vi "External interactions.vi"(10 "Message":refnum<user-event>, 11 "UUT Result":refnum<user-event>) -> ()   [LabVIEW 2025]
uses:
  Test Unit/UUT Result.ctl
  <vilib>/Test Bench Framework/Test Executive.lvlibp/TestEngine/TestEngine/TestEngine/Typedefs/Report General.ctl
  Full User Interface/Send User Message Argument--cluster.ctl
  Test Unit/Test Unit.lvlib
  Full User Interface/Full User Interface.lvlib
  <vilib>/Test Bench Framework/Test Executive.lvlibp/TestEngine/TestEngine/TestEngine/Test Engine.lvclass
panel:
  in  "Checkbox":bool
  out "当前测试型号":string
  out "General":T1
  in  "设置条码":bool
  in  "启动测试":bool
  out "Error Out":errorcluster
  in  "Error In":errorcluster
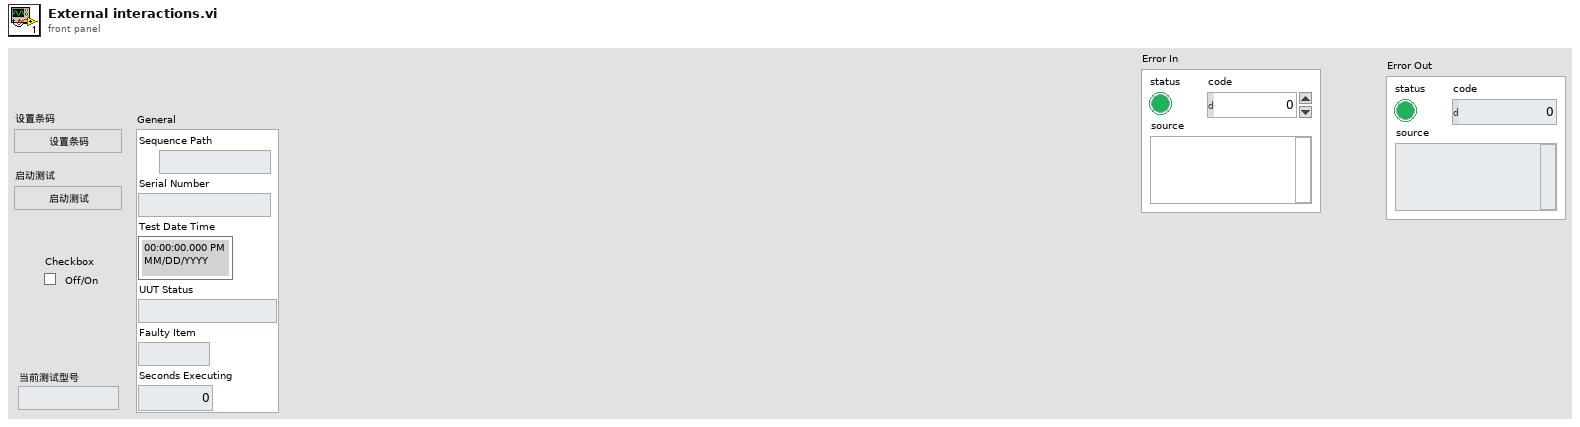
[diagram p1: front panel]
types:
  T1 = typedef "Test Executive.lvlibp/Test Engine.lvlib/Test Engine.lvclass/Report General.ctl" = cluster{"Sequence Path":path, "Serial Number":string, "Test Date Time":timestamp, "UUT Status":string, "Faulty Item":string, "Seconds Executing":dbl}
  T2 = typedef "Full User Interface.lvlib/Send User Message Argument--cluster.ctl" = cluster{"Station ID":i32, "Socket":i32, "UserMessage":string, "MessageData":variant}
  T3 = enum32{"Invalid", "Standard", "Closed", "Hidden", "Minimized", "Maximized"}
  T4 = enum32{"invalid app kind", "Development System", "Run Time System", "Student Edition", "Embedded LabVIEW", "Evaluation", "Custom"}
  T5 = cluster{"Core":cluster{"Current VI Reference":refnum<vi>, "Close Panel on Exit?":bool}, "Your Boolean data":bool, "Your string data":string}
  T6 = cluster{"Current VI Reference":refnum<vi>, "Close Panel on Exit?":bool}
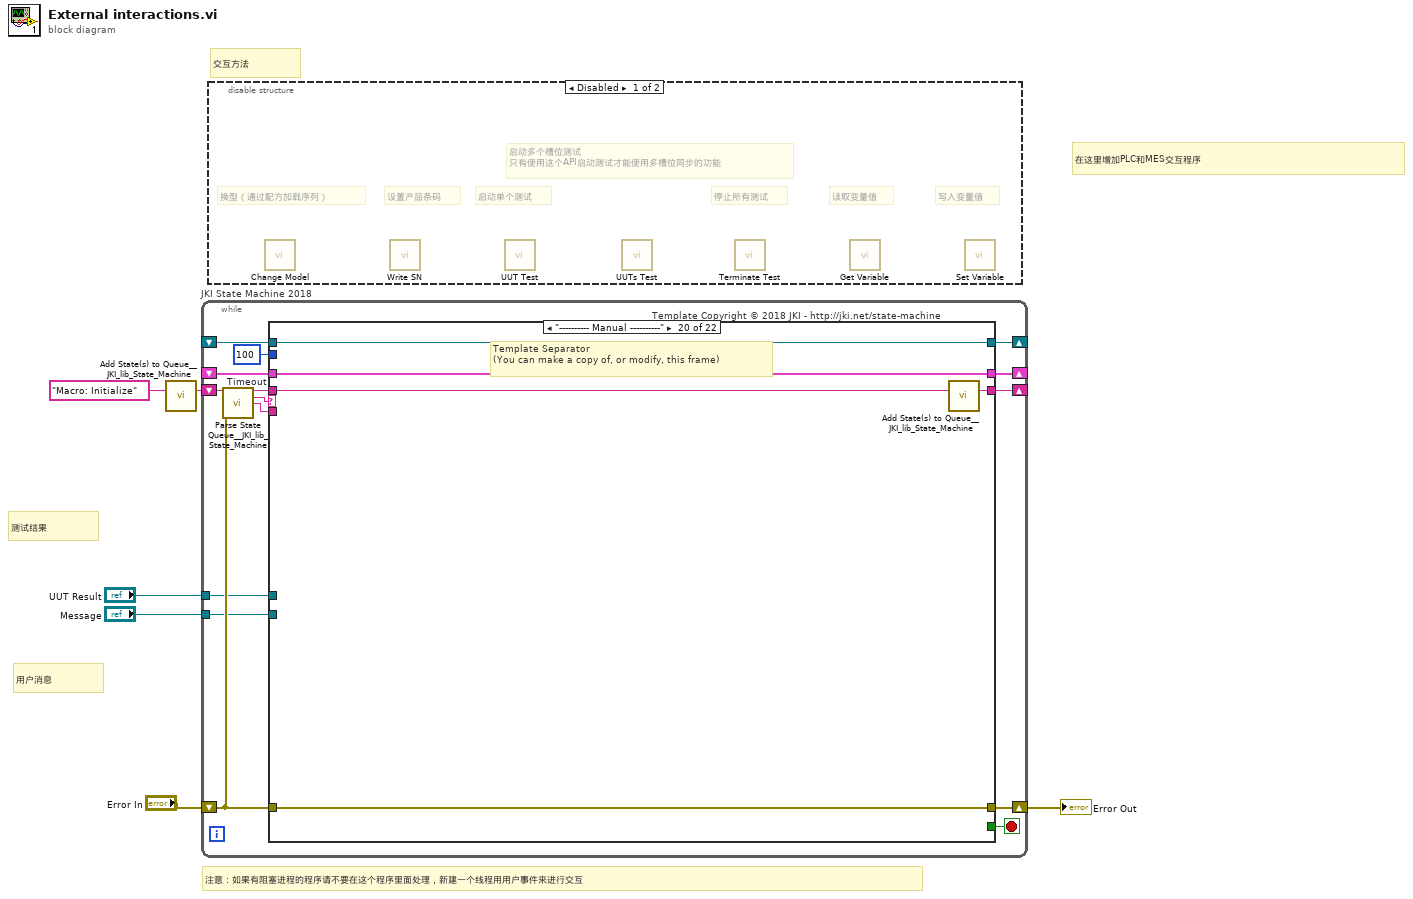
[diagram p0: block diagram]
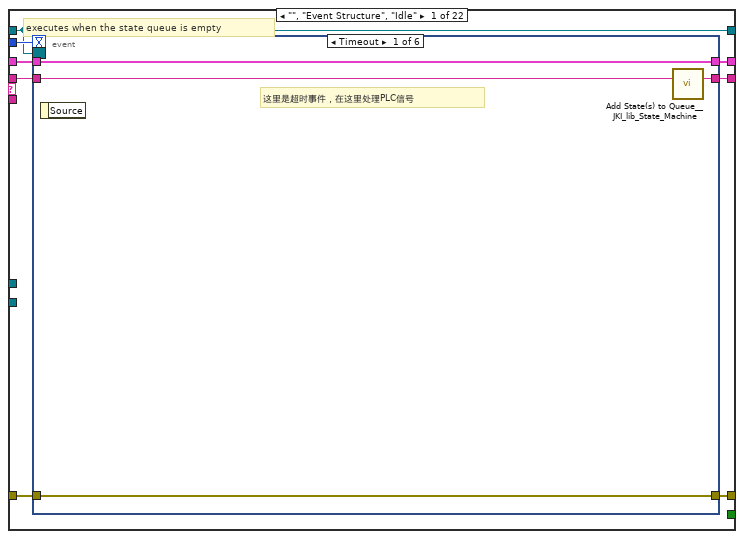
[diagram p2: hidden frame]
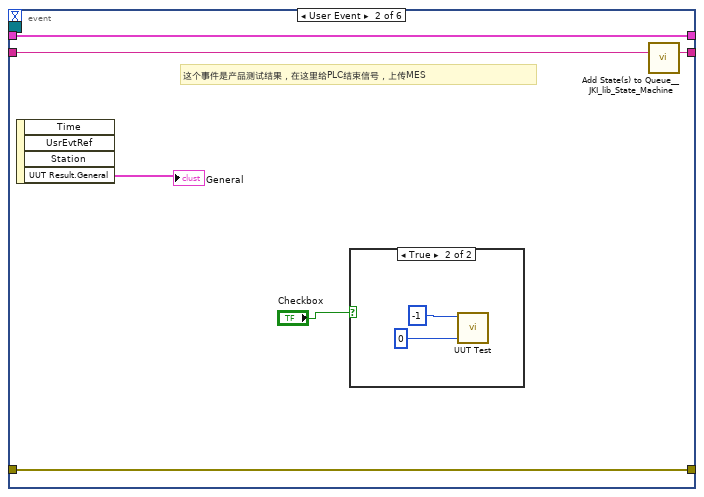
[diagram p3: hidden frame]
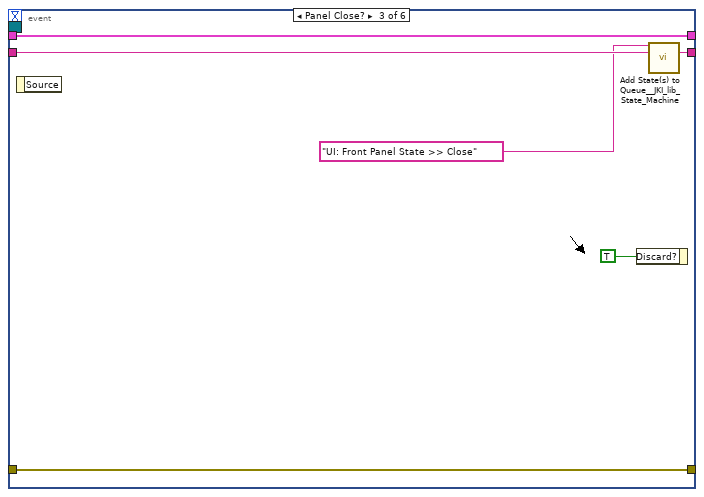
[diagram p5: hidden frame]
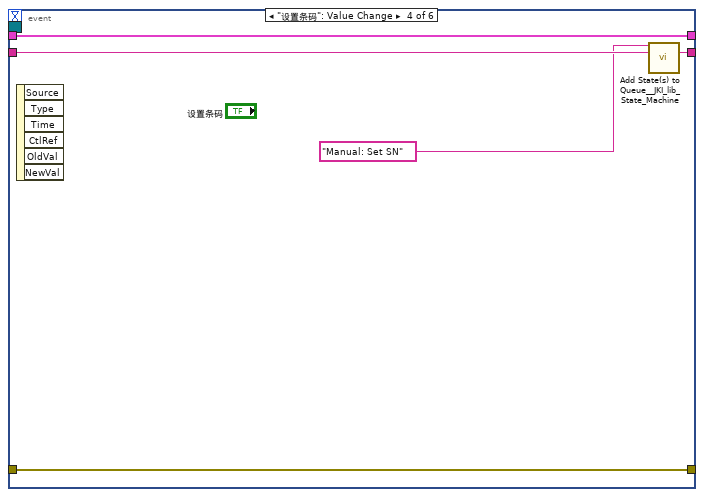
[diagram p6: hidden frame]
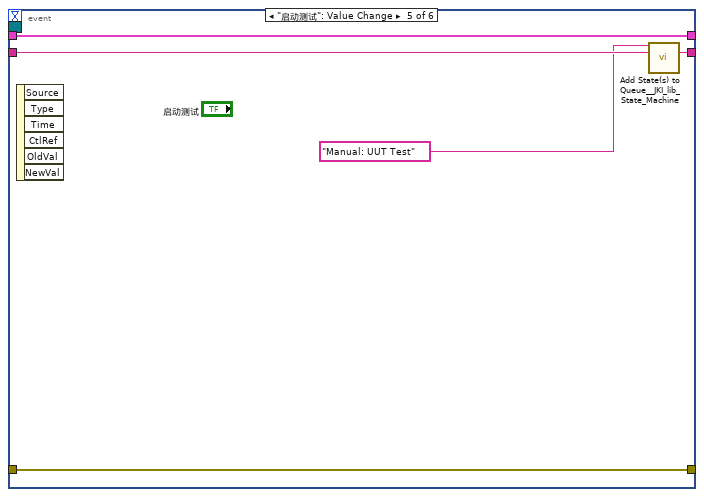
[diagram p7: hidden frame]
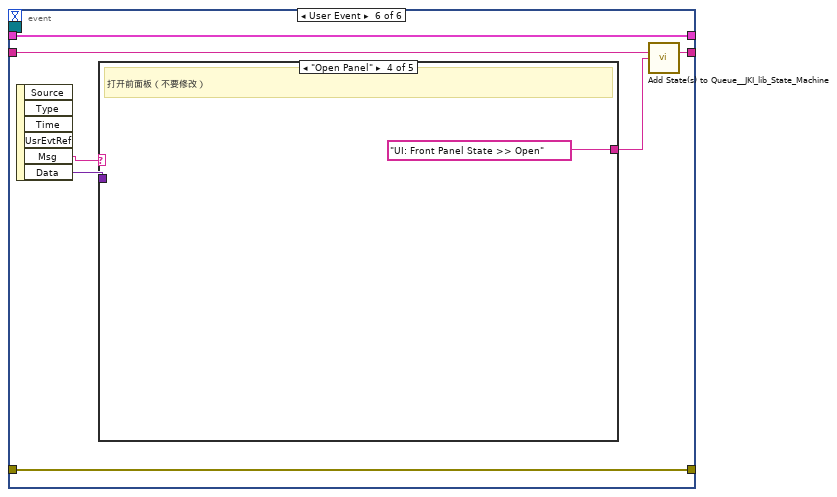
[diagram p8: hidden frame]
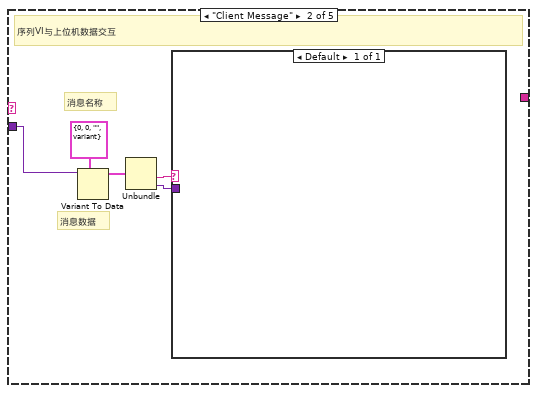
[diagram p10: hidden frame]
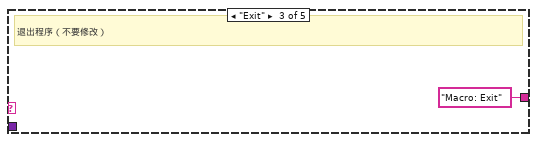
[diagram p11: hidden frame]
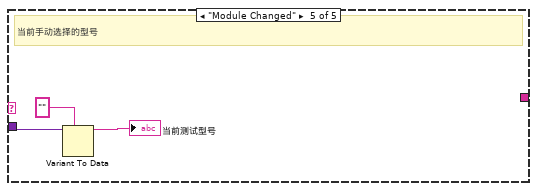
[diagram p12: hidden frame]
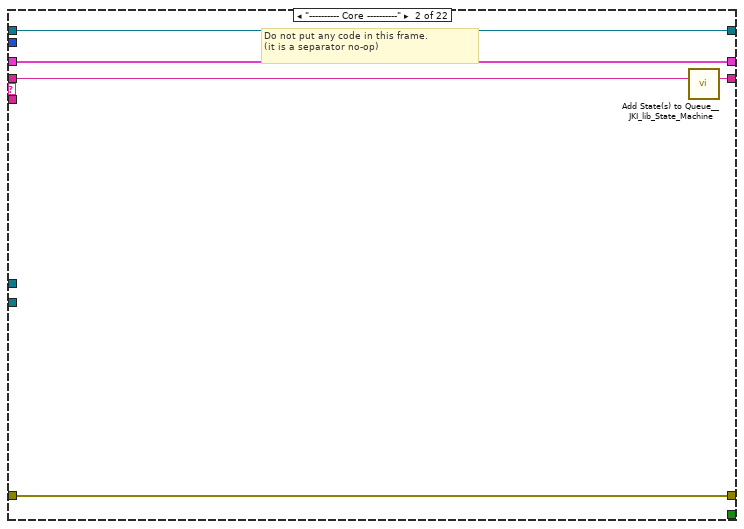
[diagram p13: hidden frame]
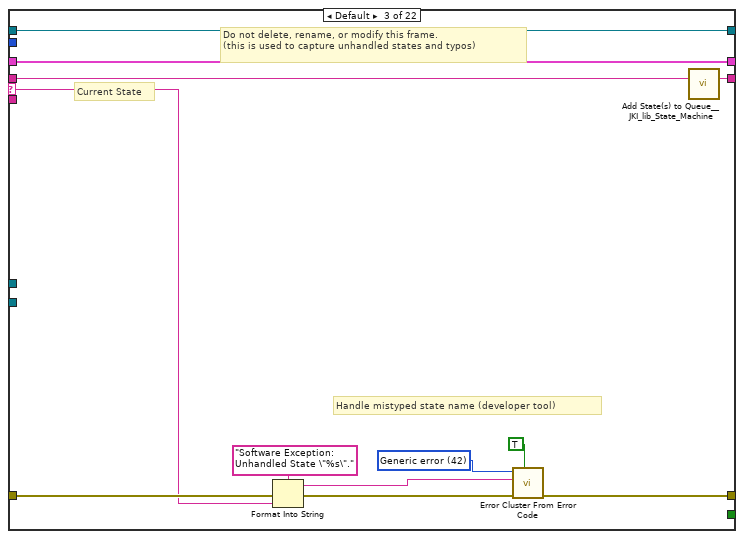
[diagram p14: hidden frame]
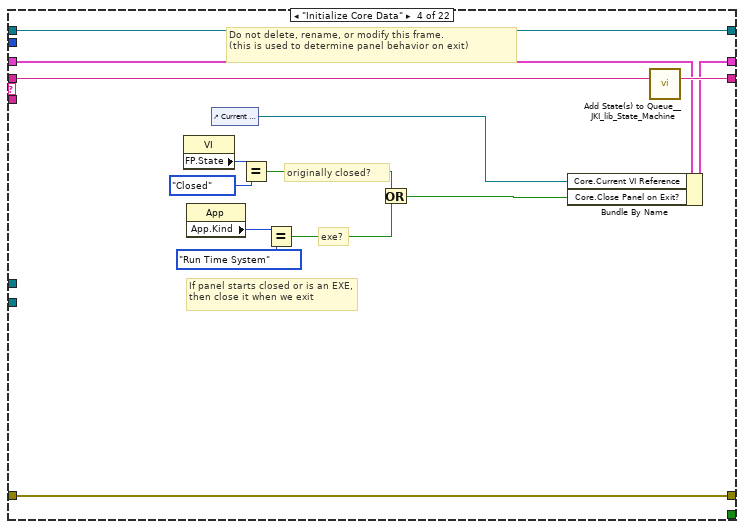
[diagram p15: hidden frame]
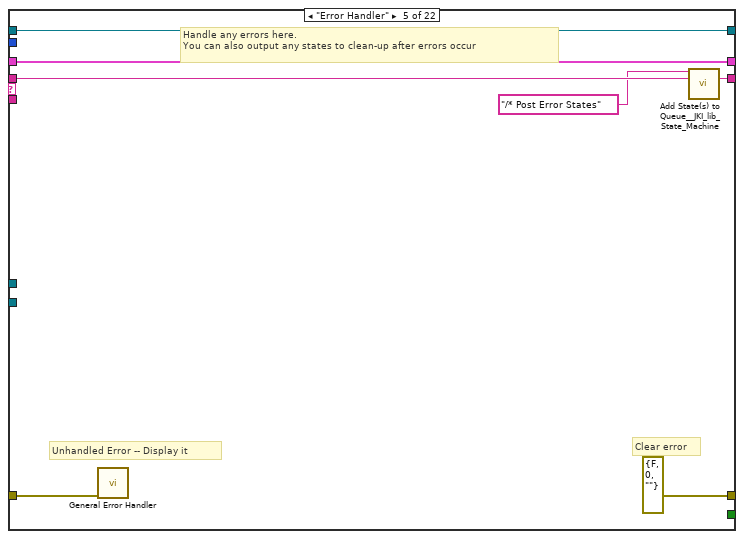
[diagram p16: hidden frame]
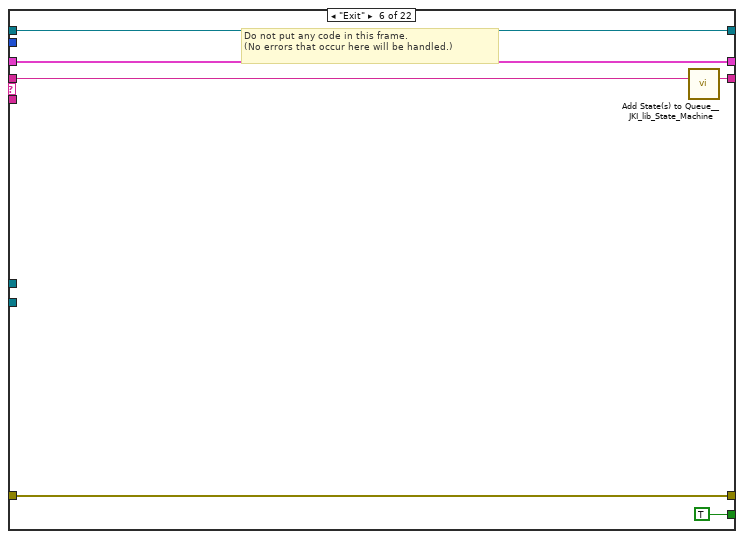
[diagram p17: hidden frame]
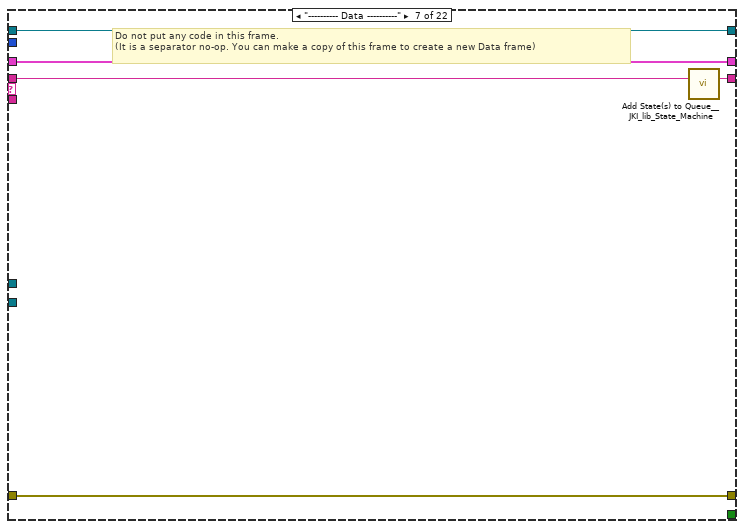
[diagram p18: hidden frame]
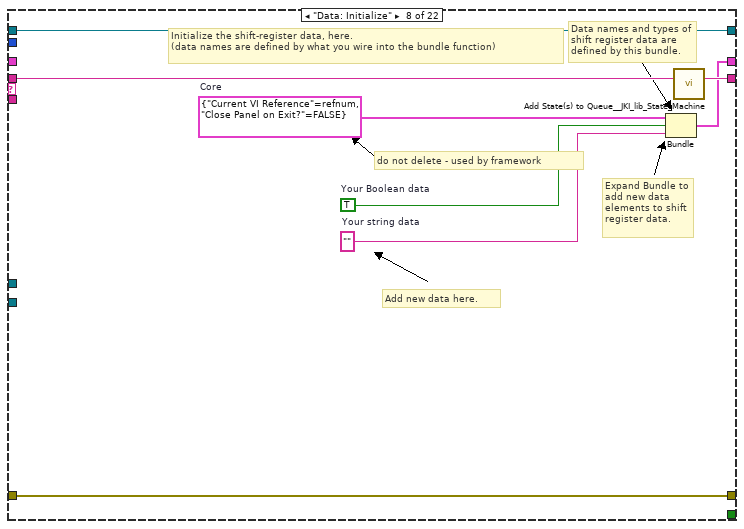
[diagram p19: hidden frame]
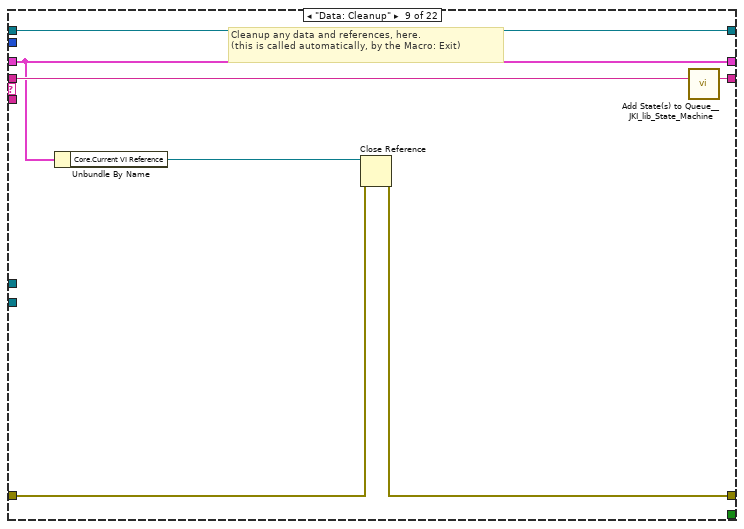
[diagram p20: hidden frame]
diagram:
  # "注意：如果有阻塞进程的程序请不要在这个程序里面处理，新建一个线程用用户事件来进行交互"
  # "在这里增加PLC和MES交互程序"
  # "用户消息"
  # "测试结果"
  # "交互方法"
  n1 = call <vilib>:"Add State(s) to Queue__JKI_lib_State_Machine.vi"("State(s) in (\"\")"="Macro: Initialize") -> ("States Out"=w6:string)  [unwired: 14 in]
  n2 = while "JKI State Machine 2018" {
    shift-right: [w14] -> _
    shift-left: _ -> [w13]
    shift-right: [w17] -> w3
    shift-left: "Error In" -> [w11]
    shift-right: [w16] -> _
    shift-left: w6 -> [w18]
    shift-right: [w10] -> _
    shift-left: _ -> [w9]
    tunnel: "UUT Result" -> [w8]
    tunnel: "Message" -> [w7]
    stop <- w15 stop-if-true
    w12 = 100  # Timeout
    # "Template Copyright © 2018 JKI - http://jki.net/state-machine"
    n3 = call <vilib>:"Parse State Queue__JKI_lib_State_Machine.vi"("State Queue"=w18, "Error In (no error)"=w11) -> ("Remaining States"=w20:string, "Current State"=w21:string, "Arguments"=w19:string)  [unwired: 11 in]
    n4 = case shown="\"---------- Manual ----------\"" w21 {
      selector: w21 -> [_ _ w81 _ _ _ _ _ _ _ _ _ _ _ _ _ _ _ _ _ _ _]
      tunnel: w20 -> [w29 w79 w85 w105 w112 w118 w123 w131 w138 w143 w151 w157 w162 w168 w175 w187 w257 w263 w274 w279 w285 w297]
      tunnel: w19 -> [_ _ _ _ _ _ _ _ _ _ _ _ _ _ w170 w181 _ _ _ _ _ _]
      tunnel: w13 -> [w27 w76 w83 w98 w109 w116 w120 _ w133 w140 w149 w155 w159 w166 w173 w183 w254 w260 w271 w276 w282 w294]
      tunnel: [w26 w77 w87 w102 errorcluster {"status"=FALSE, "code"=0, "source"=""} ("error out") w115 w121 w128 w134 w141 w147 w152 w160 w165 w171 w184 w255 w261 w272 w277 w283 w295] -> w17
      tunnel: w11 -> [w25 w77 w86 w102 w108 w115 w121 w128 w135 w141 w146 w153 w160 w165 w172 w185 w255 w261 w272 w277 w283 w295]
      tunnel: [w28 w78 w84 w104 w111 w117 w122 w130 w137 w142 w150 w156 w161 w167 w174 w186 w256 w262 w273 w278 w284 w296] -> w16
      tunnel: [_ _ _ _ _ TRUE _ _ _ _ _ _ _ _ _ _ _ _ _ _ _ _] -> w15
      tunnel: [w24 w76 w83 w103 w109 w116 w120 w129 w133 w140 w149 w155 w159 w166 w173 w183 w254 w260 w271 w276 w282 w294] -> w14
      tunnel: w12 -> [w23 _ _ _ _ _ _ _ _ _ _ _ _ _ _ _ _ _ _ _ _ _]
      tunnel: [w22 w75 w80 w92 w106 w113 w119 w124 w132 w139 w148 w154 w158 w164 w169 w180 w253 w258 w264 w275 w281 w293] -> w10
      tunnel: w9 -> [w22 w75 w80 w92 w106 w113 w119 w124 w132 w139 _ w154 w158 w164 w169 w180 w253 w258 w264 w275 w281 w293]
      tunnel: w8 -> [_ _ _ _ _ _ _ _ _ _ w145 _ _ _ _ _ _ _ _ _ _ _]
      tunnel: w7 -> [_ _ _ _ _ _ _ _ _ _ w144 _ _ _ _ _ _ _ _ _ _ _]
      frame "", "Event Structure", "Idle" {
        # "executes when the state queue is empty"
        n5 = event shown="[0] Timeout" {
          selector: w22 -> [_ _ _ _ _ _]
          dyn-events: _ -> [_ _ _ _ _ _]
          timeout: w23 -> [_ _ _ _ _ _]
          tunnel: w29 -> [w33 w39 w47 w52 w57 w64]
          tunnel: [w32 w38 w46 w51 w56 w63] -> w28
          tunnel: w27 -> [w30 w36 w44 w49 w54 w61]
          tunnel: [w31 w37 w45 w50 w55 w62] -> w26
          tunnel: w25 -> [w31 w37 w45 w50 w55 w62]
          tunnel: [w30 w36 w44 w49 w54 w61] -> w24
          event Timeout {
            # "这里是超时事件，在这里处理PLC信号"
            n6 = event-data() -> ()  [unwired: 1 in, 1 out]
            n7 = call <vilib>:"Add State(s) to Queue__JKI_lib_State_Machine.vi"("State(s) in (\"\")"=w33) -> ("States Out"=w32:string)  [unwired: 14 in]
          }
          event User Event {
            # "这个事件是产品测试结果，在这里给PLC结束信号，上传MES"
            n8 = event-data() -> ("UUT Result.General"=→"General":T1)  [unwired: 1 in, 3 out]
            n9 = case shown="True" "Checkbox" {
              frame False {
              }
              frame True {
                n10 = call "UUT Test.vi"("Socket"=0, "Station ID"=-1) -> ()  [unwired: 9 in, 1 out]
              }
            }
            n11 = call <vilib>:"Add State(s) to Queue__JKI_lib_State_Machine.vi"("State(s) in (\"\")"=w39) -> ("States Out"=w38:string)  [unwired: 14 in]
          }
          event Panel Close? {
            n12 = event-data() -> ()  [unwired: 1 in, 1 out]
            n13 = event-data("Discard?"=TRUE) -> ()  [unwired: 1 in, 1 out]
            n14 = call <vilib>:"Add State(s) to Queue__JKI_lib_State_Machine.vi"("State(s) in Front (\"\")"="UI: Front Panel State >> Close", "State(s) in (\"\")"=w47) -> ("States Out"=w46:string)  [unwired: 13 in]
          }
          event "设置条码": Value Change {
            n15 = event-data() -> ()  [unwired: 1 in, 6 out]
            n16 = call <vilib>:"Add State(s) to Queue__JKI_lib_State_Machine.vi"("State(s) in Front (\"\")"="Manual: Set SN", "State(s) in (\"\")"=w52) -> ("States Out"=w51:string)  [unwired: 13 in]
          }
          event "启动测试": Value Change {
            n17 = event-data() -> ()  [unwired: 1 in, 6 out]
            n18 = call <vilib>:"Add State(s) to Queue__JKI_lib_State_Machine.vi"("State(s) in Front (\"\")"="Manual: UUT Test", "State(s) in (\"\")"=w57) -> ("States Out"=w56:string)  [unwired: 13 in]
          }
          event User Event {
            n19 = event-data() -> ("Msg"=w60:string, "Data"=w59:variant)  [unwired: 1 in, 4 out]
            n20 = case shown="\"Open Panel\"" w60 {
              tunnel: w59 -> [_ w69 _ _ w74]
              tunnel: [_ _ "Macro: Exit" "UI: Front Panel State >> Open" _] -> w58
              frame Default {
              }
              frame "Client Message" {
                # "消息数据"
                # "消息名称"
                # "序列VI与上位机数据交互"
                n21 = Variant To Data(type=T2 {"Station ID"=0, "Socket"=0, "UserMessage"="", "MessageData"=variant(cluster{"Socket":i32, "UserMessage":string, "MessageData":variant} {"Socket"=0, "UserMessage"="", "MessageData"=variant})} ("Send User Message Argument"), Variant=w69) -> (data=w67:T2)  [unwired: 1 in, 1 out]
                n22 = Unbundle(w67) -> ("UserMessage"=w66:string, "MessageData"=w65:variant)  [unwired: 2 out]
                n23 = case shown="Default" w66 {
                  tunnel: w65 -> [_]
                  frame Default {
                  }
                }
              }
              frame "Exit" {
                # "退出程序（不要修改）"
              }
              frame "Open Panel" {
                # "打开前面板（不要修改）"
              }
              frame "Module Changed" {
                # "当前手动选择的型号"
                n24 = Variant To Data(type="", Variant=w74) -> (data=→"当前测试型号":string)  [unwired: 1 in, 1 out]
              }
            }
            n25 = call <vilib>:"Add State(s) to Queue__JKI_lib_State_Machine.vi"("State(s) in (\"\")"=w64, "State(s) at Back (\"\")"=w58) -> ("States Out"=w63:string)  [unwired: 13 in]
          }
        }
      }
      frame "---------- Core ----------" {
        # "Do not put any code in this frame.\n(it is a separator no-op)"
        n26 = call <vilib>:"Add State(s) to Queue__JKI_lib_State_Machine.vi"("State(s) in (\"\")"=w79) -> ("States Out"=w78:string)  [unwired: 14 in]
      }
      frame Default {
        w90 = 42 items=["No error", "Argument error", "Memory is full", "Out of zone", "End of file", "File already open", "Generic file I/O error", "File not found", "File permission error", "Disk is full", "Duplicate path", "Too many files open", "System feature not enabled", "Resource file not found", "Cannot add resource", "Resource not found", "Image not found", "Image memory error", "Pen does not exist", "Config type invalid", "Config token not found", "Config parse error", "Config memory error", "Bad external code format", "Bad external code offset", "External code not present", "Null window", "Destroy window error", "Null menu", "Print aborted", "Bad print record", "Print driver error", "Windows error during printing", "Memory error during printing", "Print dialog error", "Generic print error", "Invalid device refnum", "Device not found", "Device parameter error", "Device unit error", "Cannot open device", "Device call aborted", "Generic error", "Cancelled by user", "Object ID too low", "Object ID too high", "Object not in heap", "Unknown heap", "Unknown object (invalid DefProc)", "Unknown object (DefProc not in table)", "Message out of range", "Invalid (null) method", "Unknown message", "Manager call not supported", "Bad address", "Network operation in progress", "Network operation timed out", "Connection is busy", "Network attribute not supported", "Network error", "Address in use", "System out of memory", "Connection aborted", "Connection refused", "Not connected", "Already connected", "Connection closed", "Initialization error (interapplication manager)", "Bad occurrence", "Wait on unbound occurrence handler", "Occurrence queue overflow", "Datalog type conflict", "Unused", "Unrecognized type (interapplication manager)", "Memory corrupt", "Failed to make temporary DLL", "Old CIN version", "Drag socket not found", "Failed to load drop-object", "Failed to register OLE object", "Failed to release OLE object", "Format specifier type mismatch", "Unknown format specifier", "Too few format specifiers", "Too many format specifiers", "Scan failed", "Newer CIN version", "Error converting to variant", "Runtime menu error", "Password tampered", "Variant attribute not found", "Incompatible variant data type", "Event data is not available", "Event Store is not present", "Occurrence is not found", "Event Queue is not created", "Event info is not available", "Refnum passed is NULL", "Error retrieving Class GUID", "Error retrieving CoClass GUID", "Error retrieving TypeLib GUID.", "Bad built application magic bytes.", "Specific driver is different from the specific driver associated with the Logical Name.", "There is no session opened to the class driver.", "Max Error", "MAX - Error with config objects", "MAX - Error loading configuration", "MAX - Group not supported"]
        # "Current State"
        # "Do not delete, rename, or modify this frame.\n(this is used to capture unhandled states and typos)"
        # "Handle mistyped state name (developer tool)"
        n27 = Format Into String(format string="Software Exception: Unhandled State \"%s\"." ("message"), error in=w86, w81) -> (resulting string=w89:string, error out=w88:errorcluster)  [unwired: 1 in]
        n28 = call <vilib>:"Error Cluster From Error Code.vi"("show call chain? (False)"=TRUE, "error in (no error)"=w88, "error message (\"\")"=w89, "error code (0)"=w90) -> ("error out"=w87:errorcluster)  [unwired: 5 in]
        n29 = call <vilib>:"Add State(s) to Queue__JKI_lib_State_Machine.vi"("State(s) in (\"\")"=w85) -> ("States Out"=w84:string)  [unwired: 14 in]
      }
      frame "Initialize Core Data" {
        # "Do not delete, rename, or modify this frame.\n(this is used to determine panel behavior on exit)"
        # "originally closed?"
        # "exe?"
        # "If panel starts closed or is an EXE, then close it when we exit"
        n30 = property class="VI"() -> ("FP.State"=w95:T3)  [unwired: 2 in, 2 out]
        n31 = property class="App"() -> ("App.Kind"=w101:T4)  [unwired: 2 in, 2 out]
        n32 = control-ref of="Current VI Reference"() -> (w96:refnum<vi>)
        n33 = Equal?(x=w95, y=T3."Closed" ("Front Panel Window:State")) -> (x = y?=w93:bool)
        n34 = Equal?(x=w101, y=T4."Run Time System" ("Application:Kind")) -> (x = y?=w99:bool)
        n35 = Or(x=w93, y=w99) -> (x .or. y?=w97:bool)
        n36 = Bundle By Name(cluster=w98, "Core.Current VI Reference"=w96, "Core.Close Panel on Exit?"=w97) -> (w103:T5)
        n37 = call <vilib>:"Add State(s) to Queue__JKI_lib_State_Machine.vi"("State(s) in (\"\")"=w105) -> ("States Out"=w104:string)  [unwired: 14 in]
      }
      frame "Error Handler" {
        # "Unhandled Error -- Display it"
        # "Handle any errors here.\nYou can also output any states to clean-up after errors occur"
        # "Clear error"
        n38 = call <vilib>:"General Error Handler.vi"("error in (no error)"=w108) -> ()  [unwired: 10 in, 5 out]
        n39 = call <vilib>:"Add State(s) to Queue__JKI_lib_State_Machine.vi"("State(s) in Front (\"\")"="/* Post Error States", "State(s) in (\"\")"=w112) -> ("States Out"=w111:string)  [unwired: 13 in]
      }
      frame "Exit" {
        # "Do not put any code in this frame.\n(No errors that occur here will be handled.)"
        n40 = call <vilib>:"Add State(s) to Queue__JKI_lib_State_Machine.vi"("State(s) in (\"\")"=w118) -> ("States Out"=w117:string)  [unwired: 14 in]
      }
      frame "---------- Data ----------" {
        # "Do not put any code in this frame.\n(It is a separator no-op. You can make a copy of this frame to create a new Data frame)"
        n41 = call <vilib>:"Add State(s) to Queue__JKI_lib_State_Machine.vi"("State(s) in (\"\")"=w123) -> ("States Out"=w122:string)  [unwired: 14 in]
      }
      frame "Data: Initialize" {
        w125 = T6 {"Current VI Reference"=refnum, "Close Panel on Exit?"=FALSE}  # Core
        w127 = TRUE  # Your Boolean data
        w126 = ""  # Your string data
        # "do not delete - used by framework"
        # "Expand Bundle to add new data elements to shift register data."
        # "Add new data here."
        # "Data names and types of shift register data are defined by this bundle."
        # "Initialize the shift-register data, here.\n(data names are defined by what you wire into the bundle function)"
        n42 = Bundle("Core"=w125, "Your Boolean data"=w127, "Your string data"=w126) -> (w129:T5)  [unwired: 1 in]
        n43 = call <vilib>:"Add State(s) to Queue__JKI_lib_State_Machine.vi"("State(s) in (\"\")"=w131) -> ("States Out"=w130:string)  [unwired: 14 in]
      }
      frame "Data: Cleanup" {
        # "Cleanup any data and references, here.\n(this is called automatically, by the Macro: Exit)"
        n44 = Unbundle By Name(w133) -> ("Core.Current VI Reference"=w136:refnum<vi>)
        n45 = Close Reference(reference=w136, error in (no error)=w135) -> (error out=w134:errorcluster)
        n46 = call <vilib>:"Add State(s) to Queue__JKI_lib_State_Machine.vi"("State(s) in (\"\")"=w138) -> ("States Out"=w137:string)  [unwired: 14 in]
      }
      frame "---------- Events ----------" {
        # "Do not put any code in this frame.\n(It is a separator no-op. You can make a copy of this frame to create a new UI frame)"
        n47 = call <vilib>:"Add State(s) to Queue__JKI_lib_State_Machine.vi"("State(s) in (\"\")"=w143) -> ("States Out"=w142:string)  [unwired: 14 in]
      }
      frame "Events: Register" {
        # "Do not put any code in this frame.\n(It is a separator no-op. You can make a copy of this frame to create a new UI frame)"
        n48 = register-events(error in=w146, w145, w144) -> (reference out=w148:refnum<event-registration>, error out=w147:errorcluster)  [unwired: 1 in]
        n49 = call <vilib>:"Add State(s) to Queue__JKI_lib_State_Machine.vi"("State(s) in (\"\")"=w151) -> ("States Out"=w150:string)  [unwired: 14 in]
      }
      frame "Events: Unregister" {
        # "Do not put any code in this frame.\n(It is a separator no-op. You can make a copy of this frame to create a new UI frame)"
        n50 = Unregister For Events(event registration refnum=w154, error in=w153) -> (error out=w152:errorcluster)
        n51 = call <vilib>:"Add State(s) to Queue__JKI_lib_State_Machine.vi"("State(s) in (\"\")"=w157) -> ("States Out"=w156:string)  [unwired: 14 in]
      }
      frame "---------- UI ----------" {
        # "Do not put any code in this frame.\n(It is a separator no-op. You can make a copy of this frame to create a new UI frame)"
        n52 = call <vilib>:"Add State(s) to Queue__JKI_lib_State_Machine.vi"("State(s) in (\"\")"=w162) -> ("States Out"=w161:string)  [unwired: 14 in]
      }
      frame "UI: Initialize" {
        # "Initialize the User Interface, here.\n(this is called automatically, by the Macro: Init)"
        n53 = property class="VI"("Front Panel.Title"="外部交互" ("Front Panel Window:Title")) -> ()  [unwired: 2 in, 2 out]
        n54 = call <vilib>:"Add State(s) to Queue__JKI_lib_State_Machine.vi"("State(s) in (\"\")"=w168) -> ("States Out"=w167:string)  [unwired: 14 in]
      }
      frame "UI: Cursor Set" {
        # "Argument"
        # "Set and Unset Cursor Busy.\n(Usage: \"UI: Cursor Set >> Busy|Idle\")"
        n55 = case shown="\"Idle\", Default" w170 {
          tunnel: w172 -> [w177 w179]
          tunnel: [w176 w178] -> w171
          frame "Idle", Default {
            n56 = call <vilib>:"Unset Busy.vi"("error in (no error)"=w177) -> ("error out"=w176:errorcluster)  [unwired: 10 in]
          }
          frame "Busy" {
            n57 = call <vilib>:"Set Busy.vi"("error in (no error)"=w179) -> ("error out"=w178:errorcluster)  [unwired: 9 in, 1 out]
          }
        }
        n58 = call <vilib>:"Add State(s) to Queue__JKI_lib_State_Machine.vi"("State(s) in (\"\")"=w175) -> ("States Out"=w174:string)  [unwired: 14 in]
      }
      frame "UI: Front Panel State" {
        # "Argument"
        # "Set Front Panel Open or Closed\n(Usage: \"UI: Front Panel State >> Open|Close\")"
        n59 = Unbundle By Name(w183) -> ("Core.Current VI Reference"=w182:refnum<vi>)
        n60 = case shown="\"Minimize\", \"Minimized\"" w181 {
          tunnel: w185 -> [w193 w208 w219 w232 w245]
          tunnel: [w195 w209 w221 w234 w247] -> w184
          tunnel: w182 -> [w194 w206 w220 w233 w246]
          frame "Open", "Standard", Default {
            w188 = T3."Standard" ("State")
            n61 = property class="VI"(reference=w194, error in=w193) -> (reference out=w191:refnum<vi>, error out=w192:errorcluster, "FP.State"=w190:T3)
            n62 = Not Equal?(x=w190, y=w188) -> (x != y?=w189:bool)
            n63 = case shown="True" w189 {
              tunnel: [w199 w201] -> w195
              tunnel: w192 -> [w198 w201]
              tunnel: w191 -> [w197 _]
              tunnel: w188 -> [w196 _]
              frame True {
                n64 = invoke class="VI" method="FP.Open"(reference=w197, error in=w198, "Activate"=TRUE, "State"=w196) -> (error out=w199:errorcluster)  [unwired: 1 in, 4 out]
              }
              frame False {
              }
            }
          }
          frame "Close", "Closed" {
            n65 = property class="VI"(reference=w206, error in=w208) -> (reference out=w205:refnum<vi>, error out=w207:errorcluster, "FP.State"=w203:T3)
            n66 = Not Equal?(x=w203, y=T3."Closed" ("Front Panel Window:State")) -> (x != y?=w202:bool)
            n67 = case shown="True" w202 {
              tunnel: [w210 w213] -> w209
              tunnel: w207 -> [w210 w212]
              tunnel: w205 -> [_ w211]
              frame False {
              }
              frame True {
                n68 = invoke class="VI" method="FP.Close"(reference=w211, error in=w212) -> (error out=w213:errorcluster)  [unwired: 1 in, 2 out]
              }
            }
          }
          frame "Hidden", "Hide" {
            w214 = T3."Hidden" ("State")
            n69 = property class="VI"(reference=w220, error in=w219) -> (reference out=w217:refnum<vi>, error out=w218:errorcluster, "FP.State"=w216:T3)
            n70 = Not Equal?(x=w216, y=w214) -> (x != y?=w215:bool)
            n71 = case shown="True" w215 {
              tunnel: [w225 w226] -> w221
              tunnel: w218 -> [w224 w226]
              tunnel: w217 -> [w223 _]
              tunnel: w214 -> [w222 _]
              frame True {
                n72 = invoke class="VI" method="FP.Open"(reference=w223, error in=w224, "State"=w222) -> (error out=w225:errorcluster)  [unwired: 2 in, 4 out]
              }
              frame False {
              }
            }
          }
          frame "Minimize", "Minimized" {
            w227 = T3."Minimized" ("State")
            n73 = property class="VI"(reference=w233, error in=w232) -> (reference out=w230:refnum<vi>, error out=w231:errorcluster, "FP.State"=w229:T3)
            n74 = Not Equal?(x=w229, y=w227) -> (x != y?=w228:bool)
            n75 = case shown="True" w228 {
              tunnel: [w238 w239] -> w234
              tunnel: w231 -> [w237 w239]
              tunnel: w230 -> [w236 _]
              tunnel: w227 -> [w235 _]
              frame True {
                n76 = invoke class="VI" method="FP.Open"(reference=w236, error in=w237, "State"=w235) -> (error out=w238:errorcluster)  [unwired: 2 in, 4 out]
              }
              frame False {
              }
            }
          }
          frame "Maximize", "Maximized" {
            w240 = T3."Maximized" ("State")
            n77 = property class="VI"(reference=w246, error in=w245) -> (reference out=w243:refnum<vi>, error out=w244:errorcluster, "FP.State"=w242:T3)
            n78 = Not Equal?(x=w242, y=w240) -> (x != y?=w241:bool)
            n79 = case shown="True" w241 {
              tunnel: [w251 w252] -> w247
              tunnel: w244 -> [w250 w252]
              tunnel: w243 -> [w249 _]
              tunnel: w240 -> [w248 _]
              frame True {
                n80 = invoke class="VI" method="FP.Open"(reference=w249, error in=w250, "State"=w248) -> (error out=w251:errorcluster)  [unwired: 2 in, 4 out]
              }
              frame False {
              }
            }
          }
        }
        n81 = call <vilib>:"Add State(s) to Queue__JKI_lib_State_Machine.vi"("State(s) in (\"\")"=w187) -> ("States Out"=w186:string)  [unwired: 14 in]
      }
      frame "---------- Macro ----------" {
        # "Do not put any code in this frame.\n(It is a separator no-op. You can make a copy of this frame to create a new Macro frame)"
        n82 = call <vilib>:"Add State(s) to Queue__JKI_lib_State_Machine.vi"("State(s) in (\"\")"=w257) -> ("States Out"=w256:string)  [unwired: 14 in]
      }
      frame "Macro: Initialize" {
        # "Initialization Macro\n(This is called once, when the VI starts)"
        n83 = call <vilib>:"Add State(s) to Queue__JKI_lib_State_Machine.vi"("State(s) in Front (\"\")"="Data: Initialize\nInitialize Core Data\nEvents: Register\nUI: Initialize\nUI: Front Panel State >> Close", "State(s) in (\"\")"=w263) -> ("States Out"=w262:string)  [unwired: 13 in]
      }
      frame "Macro: Exit" {
        # "Exit Macro\n(This is called once, when the VI exits)"
        n84 = Unbundle By Name(w271) -> ("Core.Close Panel on Exit?"=w270:bool)
        n85 = Select(t="UI: Front Panel State >> Close", s=w270, f="") -> (s? t:f=w267:string)
        n86 = call <vilib>:"Add State(s) to Queue__JKI_lib_State_Machine.vi"("State(s) in (\"\")"=w267, "State(s) at Back (\"\")"="Data: Cleanup\nEvents: Unregister\nExit") -> ("States Out"=w265:string)  [unwired: 13 in]
        n87 = call <vilib>:"Add State(s) to Queue__JKI_lib_State_Machine.vi"("State(s) in Front (\"\")"=w265, "State(s) in (\"\")"=w274) -> ("States Out"=w273:string)  [unwired: 13 in]
      }
      frame "---------- Manual ----------" {
        # "Template Separator\n(You can make a copy of, or modify, this frame)"
        n88 = call <vilib>:"Add State(s) to Queue__JKI_lib_State_Machine.vi"("State(s) in (\"\")"=w279) -> ("States Out"=w278:string)  [unwired: 14 in]
      }
      frame "Manual: UUT Test" {
        # "Your code here.\n(You can make a copy of, or modify, this frame)"
        n89 = disable-structure shown="Enabled" {
          disable-tunnel: -1 ("Station ID") -> [w287 w289]
          frame Enabled {
            n90 = call "UUT Test.vi"("Socket"=0, "Station ID"=w287) -> ()  [unwired: 9 in, 1 out]
          }
          frame Disabled {
            n91 = call "UUTs Test.vi"("Enable Socket"=bool[] [TRUE, TRUE, TRUE, TRUE], "Station ID"=w289) -> ()  [unwired: 9 in, 1 out]
          }
        }
        n92 = call <vilib>:"Add State(s) to Queue__JKI_lib_State_Machine.vi"("State(s) in (\"\")"=w285) -> ("States Out"=w284:string)  [unwired: 14 in]
      }
      frame "Manual: Set SN" {
        # "Your code here.\n(You can make a copy of, or modify, this frame)"
        n93 = call "Write SN.vi"("Serial Number"="123", "Socket"=0, "Station ID"=-1) -> ()  [unwired: 8 in, 1 out]
        n94 = call <vilib>:"Add State(s) to Queue__JKI_lib_State_Machine.vi"("State(s) in (\"\")"=w297) -> ("States Out"=w296:string)  [unwired: 14 in]
      }
    }
  }
  "Error Out" <- w3
  n95 = disable-structure shown="Disabled" {
    frame Disabled {
      # "写入变量值"
      # "读取变量值"
      # "设置产品条码"
      # "停止所有测试"
      # "启动多个槽位测试\n只有使用这个API启动测试才能使用多槽位同步的功能"
      # "启动单个测试"
      # "换型（通过配方加载序列）"
      n96 = call "Change Model.vi"() -> ()  [unwired: 11 in, 1 out]
      n97 = call "Write SN.vi"() -> ()  [unwired: 11 in, 1 out]
      n98 = call "UUT Test.vi"() -> ()  [unwired: 11 in, 1 out]
      n99 = call "UUTs Test.vi"() -> ()  [unwired: 11 in, 1 out]
      n100 = call "Terminate Test.vi"() -> ()  [unwired: 11 in, 1 out]
      n101 = call "Get Variable.vi"() -> ()  [unwired: 7 in, 5 out]
      n102 = call "Set Variable.vi"() -> ()  [unwired: 11 in, 1 out]
    }
    frame Enabled {
    }
  }
